vi "Post-Build Action.vi"(5 "Files Generated by Build":path[](array[path]), 6 "Top Level/Always Included VIs":path[](array[path]), 7 "Destination Path":path, 8 "error in (no error)":errorcluster, 9 "Target Name":string, 10 "Build Specification Name":string, 11 "Project Path":path) -> (0 "error out":errorcluster)   [LabVIEW 2026]
doc: "This VI is called after each run of a build specification. The VI will copy the generated LLB (Engine or System Explorer) into the VeriStand Custom Device folder (...\\Documents\\National Instruments\\NI VeriStand 2013...)."
uses:
  C:/Users/ppathak/Downloads/NationalInstruments.VeriStand.dll
  Users/ppathak/Downloads/NationalInstruments.VeriStand.dll
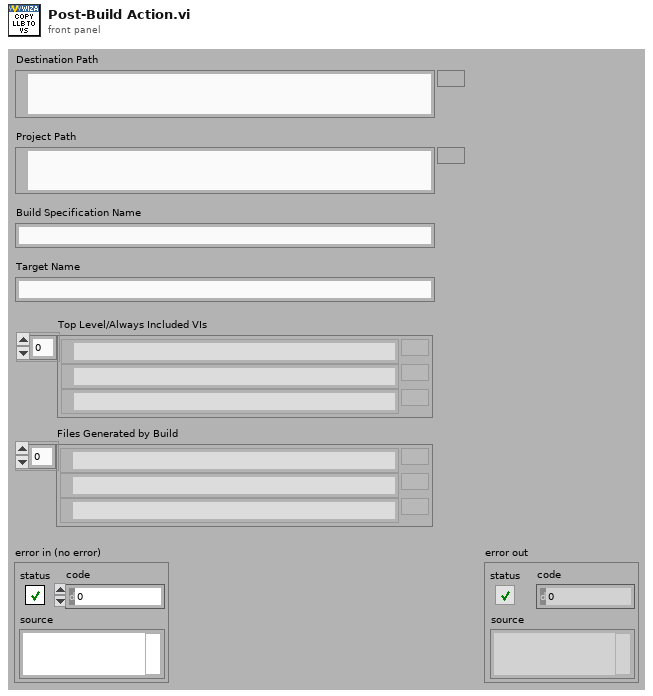
[diagram p1: front panel]
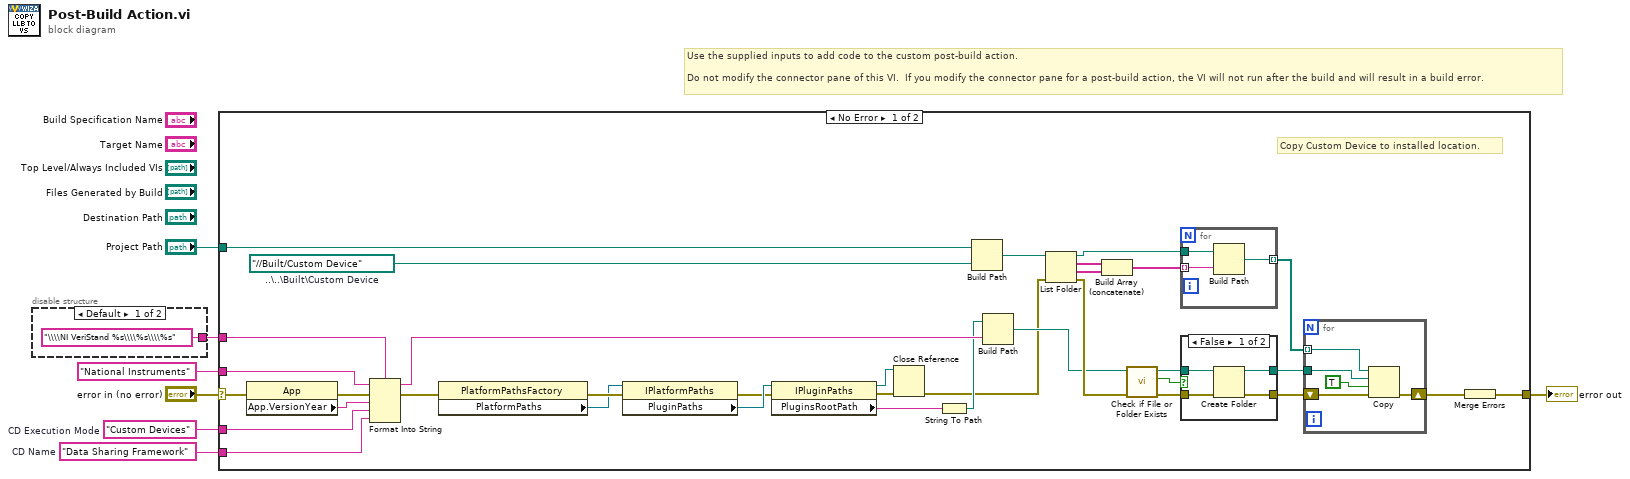
[diagram p0: block diagram]
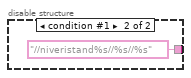
[diagram p2: hidden frame]
diagram:
  w2 = "Data Sharing Framework"  # CD Name
  w3 = "Custom Devices"  # CD Execution Mode
  # "Use the supplied inputs to add code to the custom post-build action.\n\nDo not modify the connector pane of this VI.  If you modify the connector pane for a post-build action, the VI will not run after the build and will result in a build error."
  n1 = disable-structure shown="Default" {
    disable-tunnel: ["\\\\NI VeriStand %s\\\\%s\\\\%s" ("name or relative path") "//niveristand%s//%s//%s" ("name or relative path")] -> w4
    frame condition #0 (active) {
    }
    frame condition #1 {
    }
  }
  n2 = case shown="No Error" "error in (no error)" {
    selector: "error in (no error)" -> [w31 w59]
    tunnel: [w20 w59] -> w5
    tunnel: "Project Path" -> [w26 _]
    tunnel: w4 -> [w34 _]
    tunnel: w3 -> [w33 _]
    tunnel: w2 -> [w32 _]
    tunnel: "National Instruments" ("name or relative path") -> [w29 _]
    frame No Error {
      w28 = path "../../Built/Custom Device"  # ..\..\Built\Custom Device
      # "Copy Custom Device to installed location."
      n3 = property class="App"(error in=w31) -> (error out=w36:errorcluster, "App.VersionYear"=w35:string)  [unwired: 1 in, 1 out]
      n4 = Format Into String(format string=w34, initial string=w29, error in=w36, w35, w33, w32) -> (resulting string=w37:string, error out=w11:errorcluster)
      n5 = property class="PlatformPathsFactory"(error in=w11) -> (error out=w18:errorcluster, "PlatformPaths"=w16:refnum<k24>)  [unwired: 1 in, 1 out]
      n6 = property class="IPlatformPaths"(reference=w16, error in=w18) -> (error out=w17:errorcluster, "PluginPaths"=w19:refnum<k24>)  [unwired: 1 out]
      n7 = property class="IPluginPaths"(reference=w19, error in=w17) -> (reference out=w13:refnum<k24>, error out=w14:errorcluster, "PluginsRootPath"=w15:string)
      n8 = Close Reference(reference=w13, error in (no error)=w14) -> (error out=w10:errorcluster)
      n9 = String To Path(string=w15) -> (path=w12:path)
      n10 = Build Path(base path=w26, name or relative path=w28) -> (appended path=w42:path)
      n11 = Build Path(base path=w12, name or relative path=w37) -> (appended path=w27:path)
      n12 = List Folder(path=w42, error in=w10) -> (path out=w44:path, filenames=w40:string[], folder names=w39:string[], error out=w43:errorcluster)  [unwired: 2 in]
      n13 = Build Array (concatenate)(w40, w39) -> (w38:string[])
      n14 = call <vilib>:"Check if File or Folder Exists.vi"("error in (no error)"=w43, "path"=w27) -> ("error out"=w23:errorcluster, "file or folder exists?"=w25:bool, "dup path"=w24:path)  [unwired: 7 in]
      n15 = for {
        tunnel: w38 -> [w57] mode=indexing
        tunnel: w44 -> [w58]
        tunnel: [w56] -> w30 mode=indexing
        n16 = Build Path(base path=w58, name or relative path=w57) -> (appended path=w56:path)
      }
      n17 = case shown="False" w25 {
        tunnel: w24 -> [w48 w50]
        tunnel: w23 -> [w47 w49]
        tunnel: [w46 w50] -> w22
        tunnel: [w45 w49] -> w21
        frame False {
          n18 = Create Folder(path (use dialog)=w48, error in=w47) -> (created path=w46:path, error out=w45:errorcluster)  [unwired: 1 in, 1 out]
        }
        frame True {
        }
      }
      n19 = for {
        tunnel: w30 -> [w52] mode=indexing
        shift-right: [w53] -> w41
        shift-left: w21 -> [w54]
        tunnel: w22 -> [w51]
        n20 = Copy(8:w54, 9:TRUE ("overwrite (F)"), 10:w51, 11:w52) -> (0:w53:errorcluster)  [unwired: 1 in, 2 out]
      }
      n21 = Merge Errors(w41) -> (w20:errorcluster)
    }
    frame Error {
    }
  }
  "error out" <- w5
